vi "Faraday cup Open_Close.vi"(8 "error in (no error)":errorcluster, 10 "ON/OFF":bool=TRUE, 11 "Control-Client in":refnum<class "Control-Client.lvclass">) -> (0 "error out":errorcluster, 3 "Control-Client out":refnum<class "Control-Client.lvclass">)   [LabVIEW 2020, in "Control-Client.lvclass"]
uses:
  Control-Client.lvclass
  dependecies/ControlsVIs/Clusters-def/Message types.ctl
  dependecies/ControlsVIs/Clusters-def/SERVER-Commands.ctl
  Control-Server/Control-Server.lvclass
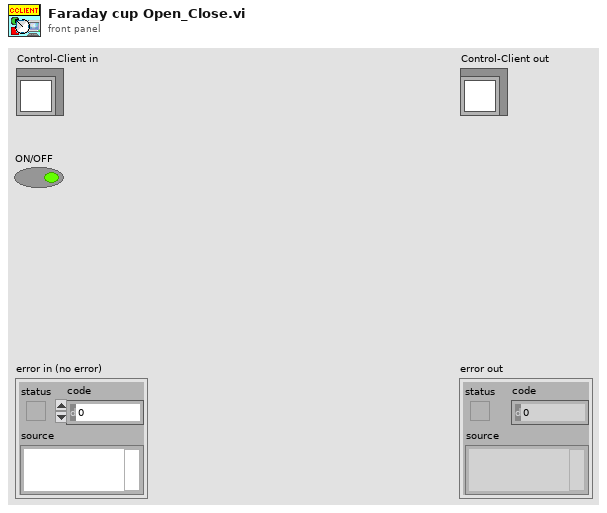
[diagram p1: front panel]
types:
  T1 = typedef "Control-Server.lvclass/SERVER-Commands.ctl" = string
  T2 = typedef "Message types.ctl" = string
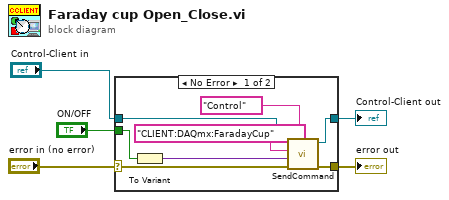
[diagram p0: block diagram]
diagram:
  n1 = case shown="No Error" "error in (no error)" {
    selector: "error in (no error)" -> [w12 w15]
    tunnel: [w11 w15] -> w4
    tunnel: [w10 w14] -> w2
    tunnel: "Control-Client in" -> [w13 w14]
    tunnel: "ON/OFF" -> [w6 _]
    frame No Error {
      n2 = To Variant(anything=w6) -> (Variant=w9:variant)
      n3 = call "SendCommand.vi"("Message type"=T2 "Control", "error in (no error)"=w12, "data"=w9, "Command"=T1 "CLIENT:DAQmx:FaradayCup" ("Commands"), "Control-Client in"=w13) -> ("error out"=w11:errorcluster, "Control-Client out"=w10:refnum<class "Control-Client.lvclass">)  [unwired: 5 in]
    }
    frame Error {
    }
  }
  "error out" <- w4
  "Control-Client out" <- w2
